vi "SR1.get start frequency.vi"(0 "i ref in":refnum<vi>, 5 "error in (no error)":errorcluster) -> (14 "i ref out":refnum<vi>, 16 "Start Frequency":dbl format="%.3f", 19 "error out":errorcluster)   [LabVIEW 2014, in "SR1.lvlib"]
doc: "reads the start frequency from the device"
uses:
  SR1.lvlib
  CSlibraries/UtilityLib/UtilityLib.valueStatus.ctl
  CS_Core/CSApplicationBaseClasses/NABase/NABase.directionType.ctl
  CS_Core/CSApplicationBaseClasses/NABase/NABase.serviceType.ctl
  CS_Core/CSSystem/CoreDefs/CoreDefs.error_type.ctl
  CS_Core/CSSystem/CoreLib/CoreLib.lvlib
  CSlibraries/UtilityLib/UtilityLib.lvlib
  instr.lib/Stanford Research SR1/Stanford Research SR1.lvlib
  CS_Core/CSApplicationBaseClasses/NABase/NABase.lvlib
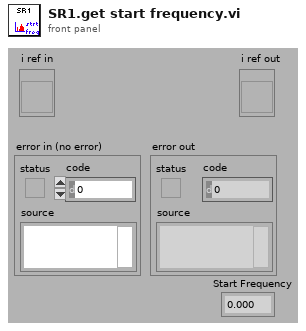
[diagram p1: front panel]
types:
  T1 = typedef "NABase.lvlib/NABase.serviceType.ctl" = enum16{"StartFreq", "NofLines", "FreqSpan", "status", "triggerLevel", "triggerSlope", "TimeRecDur", "NofStoredData"}
  T2 = typedef "NABase.lvlib/NABase.directionType.ctl" = enum16{"unknown", "update actual value", "update nominal value", "update both"}
  T3 = typedef "UtilityLib.lvlib/UtilityLib.valueStatus.ctl" = enum16{"no info available", "stand by/off", "on", "warning", "alarm/malfunction", "not implemented", "user action required", "important information", "system default", "control default", "indicator default", "button default"}
  T4 = typedef "CoreDefs.error_type.ctl" = enum16{"no error", "can't load process", "can't unload process", "process does not exist", "can't install process", "can't remove process", "unknown function", "time out", "can't execute function", "duplicate queue name", "super not found", "caller queue invalid", "can't ping process", "unknown error", "VISA Error", "VISA timeout", "GPIB timeout", "GPIB error", "communication error", "data type mismatch", "can't read data from OPC server", "can't write data to OPC server", "OET error", "function not implemented", "process already exists", "invalid Shared Variable name", "error writing Shared Variable", "error reading Shared Variable", "invalid client name", "corrupt database", "unknown class", "call not authorized", "parameter out of range", "OET timeout: can't get data to modify", "invalid queue name", "requested operation incompatible with current state", "event undefined", "event disabled", "state undefined", "caller is not a friend", "EventBuilder: bad eventID", "EventBuilder: no DAQ devices", "a thread must not stop itself", "UNUSED ELEMENT4", "DiscArchiver: eventData incomplete", "DiscArchiver: eventData does not belong to run", "DiscArchiver: can't open file", "DiscArchiver: can't write to file", "DiscArchiver: available disc space low", "can't acquire semaphore", "error reading data from database", "notifier object is not existing", "can't register process", "can't unregister process", "illegal event type", "object disabled", "object already exists", "can't change state", "Instrument not found", "no connection to remote node", "invalid reference", "N/A", "UNUSED ELEMENT 1", "element not found", "illegal TCP/IP connection detected", "object does not exist", "invalid access ID", "unknown CS system", "invalid privilige", "unsupported data type", "unsupported server type", "IO server already exists", "Shared Variable already exists"}
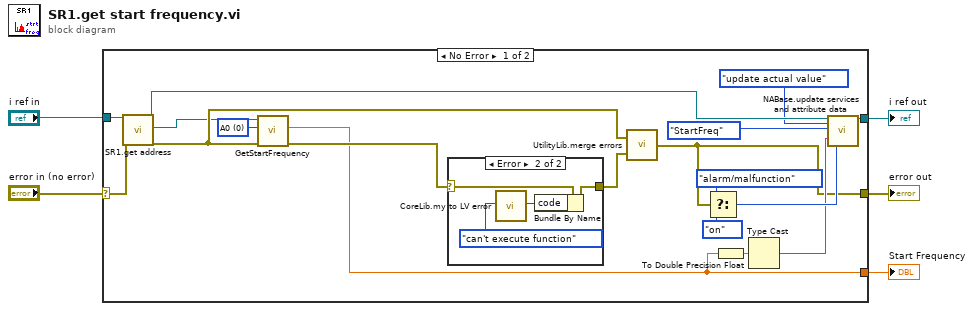
[diagram p0: block diagram]
diagram:
  n1 = case shown="No Error" "error in (no error)" {
    selector: "error in (no error)" -> [w21 w30]
    tunnel: "i ref in" -> [w23 w29]
    tunnel: [w13 w30] -> w4
    tunnel: [w14 w29] -> w3
    tunnel: [w9 _] -> w2
    frame No Error {
      w8 = 0 items=["A0", "A1"] ("Analyzer (0: A0)")
      n2 = call "SR1.get address.vi"("i ref in"=w23, "error in (no error)"=w21) -> ("i ref out"=w15:refnum<vi>, "VISA resource name"=w11:refnum<visa-resource-name>, "error out"=w12:errorcluster)  [unwired: 15 in]
      n3 = call "GetStartFrequency.vi"("error in (no error)"=w12, "Analyzer (0: A0)"=w8, "VISA resource name"=w11) -> ("error out"=w10:errorcluster, "Start Frequency [Hz]"=w9:dbl)  [unwired: 6 in, 1 out]
      n4 = case shown="Error" w10 {
        selector: w10 -> [w24 w28]
        tunnel: [w24 w25] -> w22
        frame No Error {
        }
        frame Error {
          n5 = call "CoreLib.my to LV error.vi"("ErrorTypes"=CoreDefs.error_type."can't execute function") -> ("LV error code"=w27:i32)  [unwired: 17 in, 1 out]
          n6 = Bundle By Name(cluster=w28, "code"=w27) -> (w25:errorcluster)
        }
      }
      n7 = call "UtilityLib.merge errors.vi"("error2 (no error)"=w22, "error1 (no error)"=w12) -> ("error out"=w13:errorcluster)
      n8 = Select(t=UtilityLib.valueStatus."alarm/malfunction" ("quality"), s=w13, f=UtilityLib.valueStatus."on") -> (s? t:f=w18:T3)
      n9 = To Double Precision Float(number=w9) -> (double precision float=w16:dbl)
      n10 = Type Cast(x=w16) -> (*(type *) &x=w17:string)  [unwired: 1 in]
      n11 = call "NABase.update services and attribute data.vi"("i ref in"=w15, "direction"=NABase.directionType."update actual value", "service"=NABase.serviceType."StartFreq", "value"=w17, "quality"=w18) -> ("i ref out"=w14:refnum<vi>)  [unwired: 12 in, 2 out]
    }
    frame Error {
    }
  }
  "error out" <- w4
  "i ref out" <- w3
  "Start Frequency" <- w2
